vi "Main Tclk.vi"() -> ()   [LabVIEW 2018] (continued)
            n4337 = Index Array(array=w3502) -> (element #1=w3500:i32, element #2=w3499:i32)  [unwired: 2 in]
            n4338 = Bundle By Name(cluster=w3506, "Y stig"=w3501, "X tiles"=w3499, "Y tiles"=w3500) -> (w3505:T26)
            n4339 = local write "SEM Scan Parameters"(w3505) -> ()
          }
          event "SEM Scan Parameters.X aln": Mouse Down; "SEM Scan Parameters.X aln": Value Change {
            n4340 = event-data() -> ()  [unwired: 5 out]
            n4341 = local read "SEM Scan Parameters"() -> (w3518:T26)
            n4342 = Unbundle By Name(w3518) -> ("X aln"=w3520:sgl[][], "X tiles"=w3516:u8, "Y tiles"=w3515:u8)
            n4343 = call "2D array edit.vi"("Data Entry Limits:Increment"=0.1, "Display Format:Precision"=u8 2, "Rows"=w3515, "Columns"=w3516, "Caption.Text"="X aln (%)", "Input array"=w3520) -> ("Output array"=w3513:sgl[][])  [unwired: 5 in]
            n4344 = Array Size(array=w3513) -> (size(s)=w3514:i32[])
            n4345 = Index Array(array=w3514) -> (element #1=w3512:i32, element #2=w3511:i32)  [unwired: 2 in]
            n4346 = Bundle By Name(cluster=w3518, "X aln"=w3513, "X tiles"=w3511, "Y tiles"=w3512) -> (w3517:T26)
            n4347 = local write "SEM Scan Parameters"(w3517) -> ()
          }
          event "SEM Scan Parameters.Y aln": Mouse Down; "SEM Scan Parameters.Y aln": Value Change {
            n4348 = event-data() -> ()  [unwired: 5 out]
            n4349 = local read "SEM Scan Parameters"() -> (w3530:T26)
            n4350 = Unbundle By Name(w3530) -> ("Y aln"=w3532:sgl[][], "X tiles"=w3528:u8, "Y tiles"=w3527:u8)
            n4351 = call "2D array edit.vi"("Data Entry Limits:Increment"=0.1, "Display Format:Precision"=u8 2, "Rows"=w3527, "Columns"=w3528, "Caption.Text"="Y aln (%)", "Input array"=w3532) -> ("Output array"=w3525:sgl[][])  [unwired: 5 in]
            n4352 = Array Size(array=w3525) -> (size(s)=w3526:i32[])
            n4353 = Index Array(array=w3526) -> (element #1=w3523:i32, element #2=w3524:i32)  [unwired: 2 in]
            n4354 = Bundle By Name(cluster=w3530, "Y aln"=w3525, "X tiles"=w3524, "Y tiles"=w3523) -> (w3529:T26)
            n4355 = local write "SEM Scan Parameters"(w3529) -> ()
          }
          event "SEM Scan Parameters.dX (um)": Mouse Down {
            w3535 = u8 1 ("Rows")
            n4356 = event-data() -> ()  [unwired: 9 out]
            n4357 = local read "SEM Scan Parameters"() -> (w3543:T26)
            n4358 = local write "Delta X array for stop limit"(sgl[] [] ("Delta X array for stop limit")) -> ()
            n4359 = Unbundle By Name(w3543) -> ("dX (um)"=w3539:sgl[], "Y tiles"=w3534:u8)
            n4360 = Reshape Array(w3539, w3534, w3535) -> (w3538:sgl[][])
            n4361 = call "2D array edit.vi"("Data Entry Limits:Increment"=0.1, "Display Format:Precision"=u8 2, "Rows"=w3534, "Columns"=w3535, "Caption.Text"="dX (um)", "Input array"=w3538) -> ("Output array"=w3537:sgl[][])  [unwired: 5 in]
            n4362 = Reshape Array(w3537, w3534) -> (w3536:sgl[])
            n4363 = Bundle By Name(cluster=w3543, "dX (um)"=w3536, "Y tiles"=w3534) -> (w3542:T26)
            n4364 = local write "SEM Scan Parameters"(w3542) -> ()
          }
          event "SEM Scan Parameters.dY (um)": Mouse Down {
            w3550 = u8 1 ("Rows")
            n4365 = event-data() -> ()  [unwired: 9 out]
            n4366 = local read "SEM Scan Parameters"() -> (w3555:T26)
            n4367 = local write "Delta Y array for stop limit"(sgl[] [] ("Delta X array for stop limit")) -> ()
            n4368 = Unbundle By Name(w3555) -> ("dY (um)"=w3551:sgl[], "X tiles"=w3546:u8)
            n4369 = Reshape Array(w3551, w3550, w3546) -> (w3549:sgl[][])
            n4370 = call "2D array edit.vi"("Data Entry Limits:Increment"=0.1, "Display Format:Precision"=u8 2, "Rows"=w3550, "Columns"=w3546, "Caption.Text"="dY (um)", "Input array"=w3549) -> ("Output array"=w3548:sgl[][])  [unwired: 5 in]
            n4371 = Reshape Array(w3548, w3546) -> (w3547:sgl[])
            n4372 = Bundle By Name(cluster=w3555, "dY (um)"=w3547, "X tiles"=w3546) -> (w3554:T26)
            n4373 = local write "SEM Scan Parameters"(w3554) -> ()
          }
          event "Mid Mag SEM": Value Change {
            n4374 = event-data() -> ()  [unwired: 6 out]
          }
          event "Mill Manual Pause": Value Change {
            w3562 = u8 0 ("AF Count")
            w3564 = FALSE ("Reset WD")
            w3563 = TRUE ("Reset WD")
            n4375 = event-data() -> ("NewVal"=w3565:bool)  [unwired: 5 out]
            n4376 = case shown="False" w3565 {
              frame False {
                n4377 = local read "Status message"() -> (w3571:string)
                n4378 = Equal?(x=w3571, y="Manual pausing ..." ("Status message")) -> (x = y?=w3570:bool)
                n4379 = Select(t="SEM between FIB" ("Status message"), s=w3570, f="Resume FIB milling ..." ("Status message")) -> (s? t:f=w3569:string)
                n4380 = local write "Status message"(w3569) -> ()
              }
              frame True {
                n4381 = local read "Status message"() -> (w3577:string)
                n4382 = Equal?(x=w3577, y="SEM between FIB" ("Status message")) -> (x = y?=w3574:bool)
                n4383 = Select(t="Manual pausing ..." ("Status message"), s=w3574, f="Manual paused" ("Status message")) -> (s? t:f=w3573:string)
                n4384 = local write "Status message"(w3573) -> ()
              }
            }
            n4385 = local write "SW error warning armed"(w3563) -> ()
            n4386 = local write "Auto Focus"(w3564) -> ()
            n4387 = local write "Auto Stig"(w3564) -> ()
            n4388 = local write "Auto Align"(w3564) -> ()
            n4389 = local write "Reset Focus"(w3563) -> ()
            n4390 = local write "3D image paused armed"(w3563) -> ()
            n4391 = local write "Temperature warning armed"(w3563) -> ()
            n4392 = local write "AF Count"(w3562) -> ()
            n4393 = local write "AS Count"(w3562) -> ()
            n4394 = local write "AA Count"(w3562) -> ()
            n4395 = local read "SEM Scan Parameters"() -> (w3558:T26)
            n4396 = Unbundle By Name(w3558) -> ("Y tiles"=w3559:u8, "X tiles"=w3560:u8)
            n4397 = Initialize Array(FALSE ("ASX Success"), w3559, w3560) -> (w3561:bool[][])
            n4398 = local write "AAY Success tiled"(w3561) -> ()
            n4399 = local write "AF Success tiled"(w3561) -> ()
            n4400 = local write "ASX Success tiled"(w3561) -> ()
            n4401 = local write "ASY Success tiled"(w3561) -> ()
            n4402 = local write "AAX Success tiled"(w3561) -> ()
          }
          event "Save Probe Table": Value Change {
            n4403 = event-data() -> ("NewVal"=w3578:bool)  [unwired: 5 out]
            n4404 = case shown="True" w3578 {
              frame False {
              }
              frame True {
                n4405 = Two Button Dialog(message="Save FIB Probe Table?") -> (T button?=w3579:bool)  [unwired: 2 in]
                n4406 = case shown="True" w3579 {
                  frame False {
                    n4407 = local write "Save Probe Table"(FALSE ("Min FIB probe")) -> ()
                  }
                  frame True {
                    n4408 = stacked-sequence {
                      frame #0 {
                        n4409 = local read "Api"() -> (w3583:refnum<k7>)
                        n4410 = local read "FIB Milling Probe"() -> (w3582:string)
                        n4411 = call "SmartSEM Remote API save FIB probe table.vi"("FIB Probe"=w3582, "Api"=w3583) -> ()  [unwired: 8 in, 2 out]
                        n4412 = local write "Status message"("Measuring FIB probe currents" ("Status message")) -> ()
                      }
                      frame #1 {
                        n4413 = local write "Save Probe Table"(FALSE ("Min FIB probe")) -> ()
                        n4414 = local write "Status message"("FIB Probe Table saved" ("Status message")) -> ()
                      }
                    }
                  }
                }
              }
            }
          }
          event "FIB Milling Probe": Value Change {
            n4415 = event-data() -> ()  [unwired: 6 out]
            n4416 = local read "Machine Type"() -> (w3587:u8)
            n4417 = case shown="2" w3587 {
              frame 0, Default {
              }
              frame 2 {
                n4418 = local read "Api"() -> (w3594:refnum<k7>)
                n4419 = call "SmartSEM Remote API set string.vi"("vValue"="FIB Milling Probe", "lpszParam"="DP_FIB_IMAGE_PROBE", "Api"=w3594) -> ("error out"=w3588:errorcluster, "Api out"=w3591:refnum<k7>)  [unwired: 7 in]
                n4420 = call "SmartSEM Remote API set string.vi"("error in"=w3588, "vValue"="Undefined", "lpszParam"="DP_FIB_MILL_PROBE", "Api"=w3591) -> ()  [unwired: 6 in, 2 out]
              }
            }
          }
          event "Min FIB probe": Value Change {
            n4421 = event-data() -> ("NewVal"=w3595:bool)  [unwired: 5 out]
            n4422 = case shown="True" w3595 {
              frame False {
              }
              frame True {
                n4423 = Two Button Dialog(message="Switch to min current of the same probe size?") -> (T button?=w3596:bool)  [unwired: 2 in]
                n4424 = case shown="True" w3596 {
                  frame False {
                    n4425 = local write "Min FIB probe"(FALSE ("Min FIB probe")) -> ()
                  }
                  frame True {
                    n4426 = stacked-sequence {
                      frame #0 {
                        n4427 = local read "Api"() -> (w3601:refnum<k7>)
                        n4428 = local read "FIB Milling Probe"() -> (w3602:string)
                        n4429 = local write "Min FIB probe"(FALSE ("Min FIB probe")) -> ()
                        n4430 = call "SmartSEM Remote API goto min or max FIB probe current.vi"("Min or Max"="Min", "FIB Probe"=w3602, "Api"=w3601) -> ("Goto probe"=w3599:string)  [unwired: 7 in, 1 out]
                        n4431 = local write "FIB Milling Probe"(w3599) -> ()
                        n4432 = local write "Status message"("Measuring FIB probe currents" ("Status message")) -> ()
                      }
                      frame #1 {
                        n4433 = local write "Status message"("Switched to minimal current of the same probe" ("Status message")) -> ()
                      }
                    }
                  }
                }
              }
            }
          }
          event "Max FIB probe": Value Change {
            n4434 = event-data() -> ("NewVal"=w3606:bool)  [unwired: 5 out]
            n4435 = case shown="True" w3606 {
              frame False {
              }
              frame True {
                n4436 = Two Button Dialog(message="Switch to max current of the same probe size?") -> (T button?=w3607:bool)  [unwired: 2 in]
                n4437 = case shown="True" w3607 {
                  frame False {
                    n4438 = local write "Max FIB probe"(FALSE ("Min FIB probe")) -> ()
                  }
                  frame True {
                    n4439 = stacked-sequence {
                      frame #0 {
                        n4440 = local read "Api"() -> (w3613:refnum<k7>)
                        n4441 = local read "FIB Milling Probe"() -> (w3612:string)
                        n4442 = local write "Max FIB probe"(FALSE ("Min FIB probe")) -> ()
                        n4443 = call "SmartSEM Remote API goto min or max FIB probe current.vi"("Min or Max"="Max", "FIB Probe"=w3612, "Api"=w3613) -> ("Goto probe"=w3611:string)  [unwired: 7 in, 1 out]
                        n4444 = local write "FIB Milling Probe"(w3611) -> ()
                        n4445 = local write "Status message"("Measuring FIB probe currents" ("Status message")) -> ()
                      }
                      frame #1 {
                        n4446 = local write "Status message"("Switched to maximal current of the same probe" ("Status message")) -> ()
                      }
                    }
                  }
                }
              }
            }
          }
          event "FIB time lapse": Value Change {
            n4447 = event-data() -> ("NewVal"=w3617:bool)  [unwired: 5 out]
            n4448 = case shown="False" w3617 {
              frame False {
                n4449 = stacked-sequence {
                  frame #0 {
                    n4450 = local read "FIB HW Config"() -> (w3620:T23)
                    n4451 = Unbundle By Name(w3620) -> ("Beam blank"=w3621:tag)
                    n4452 = local read "Api"() -> (w3618:refnum<k7>)
                    n4453 = call "FIB beam blank.vi"("Api"=w3618, "Beam blanked"=TRUE ("Ext on"), "lines"=w3621) -> ()  [unwired: 2 in, 1 out]
                  }
                  frame #1 {
                    n4454 = local read "SEM HW Config"() -> (w3626:T9)
                    n4455 = Unbundle By Name(w3626) -> ("Detector FIB-NI auto switch"=w3627:tag)
                    n4456 = call-poly <vilib>:"DAQmx Create Virtual Channel.vi"("lines"=w3627) -> ("task out"=w3624:refnum<k21>, "error out"=w3625:errorcluster)  [unwired: 4 in, 9 out]
                    n4457 = call-poly <vilib>:"DAQmx Write.vi"("task/channels in"=w3624, "data"=FALSE, "error in"=w3625) -> ("task out"=w3622:refnum<k21>, "error out"=w3623:errorcluster)  [unwired: 1 in, 10 out]
                    n4458 = call <vilib>:"DAQmx Clear Task.vi"("task in"=w3622, "error in"=w3623) -> ()  [unwired: 14 out]
                  }
                  frame #2 {
                    n4459 = local read "FIB HW Config"() -> (w3631:T23)
                    n4460 = Unbundle By Name(w3631) -> ("FIB Ext Scan"=w3630:tag)
                    n4461 = call "FIB ext scan.vi"("Ext on"=FALSE, "FIB Ext Scan"=w3630) -> ()  [unwired: 9 in, 1 out]
                  }
                  frame #3 {
                    n4462 = local read "Machine Type"() -> (w3632:u8)
                    n4463 = case shown="2" w3632 {
                      frame 0, Default {
                      }
                      frame 1 {
                        w3633 = TRUE ("Initialization")
                        n4464 = local read "COM port"() -> (w3639:refnum<visa-resource-name>)
                        n4465 = call "FIB mode.vi"("Initialization"=w3633, "FIB mode"=T10."SEM", "COM port in"=w3639) -> ("COM port out"=w3638:refnum<visa-resource-name>)  [unwired: 7 in, 1 out]
                        n4466 = call "Remcon32 command.vi"("SEM command"="edx 0", "COM port in"=w3638) -> ("COM port out"=w3637:refnum<visa-resource-name>)  [unwired: 6 in, 3 out]
                        n4467 = call "Remcon32 command.vi"("Close session"=w3633, "SEM command"="frez", "COM port in"=w3637) -> ()  [unwired: 5 in, 4 out]
                      }
                      frame 2 {
                        n4468 = local read "Api"() -> (w3640:refnum<k7>)
                        n4469 = call "SmartSEM Remote API set float.vi"("vValue"=sgl 2.0, "lpszParam"="DP_FIB_BLANKER_MODE" ("lpszCommand"), "Api"=w3640) -> ("error out"=w3641:errorcluster, "Api out"=w3642:refnum<k7>)  [unwired: 7 in]
                        n4470 = call "SmartSEM Remote API FIB mode.vi"("error in"=w3641, "FIB mode"=T50."SEM", "Api"=w3642) -> ("error out"=w3645:errorcluster, "Api out"=w3646:refnum<k7>)  [unwired: 7 in]
                        n4471 = invoke class="_EMApi" method="Execute"(reference=w3646, error in=w3645, "lpszCommand"="CMD_FREEZE_ALL") -> ()  [unwired: 1 in, 4 out]
                      }
                    }
                  }
                  frame #4 {
                    n4472 = local write "Status message"("standby" ("Status message")) -> ()
                  }
                }
              }
              frame True {
              }
            }
          }
          event "FIB Image": Mouse Down {
            n4473 = event-data() -> ("Coords"=→"Mouse Down Coords":T22)  [unwired: 3 out]
            n4474 = register-events(reference=w3658, w3654) -> (reference out=w3657:refnum<event-registration>, error out=w3656:errorcluster)  [unwired: 1 in]
            n4475 = local read "Spot"() -> (w3653:bool)
            n4476 = property on="Cursor Z (V)" class="DigNum (strict)"("Visible"=FALSE) -> ()  [unwired: 2 in, 2 out]
            n4477 = case shown="True" w3653 {
              frame False {
              }
              frame True {
                n4478 = local read "FIB HW Config"() -> (w3662:T23)
                n4479 = Unbundle By Name(w3662) -> ("Beam blank"=w3661:tag)
                n4480 = local read "Api"() -> (w3659:refnum<k7>)
                n4481 = call "FIB beam blank.vi"("Api"=w3659, "Beam blanked"=TRUE, "lines"=w3661) -> ()  [unwired: 2 in, 1 out]
              }
            }
            "Mouse down" <- TRUE ("Mouse down")
          }
          event "FIB Image": Mouse Move {
            n4482 = event-data() -> ("Coords"=w3667:T22)  [unwired: 1 out]
            n4483 = local read "Mouse down"() -> (w3666:bool)
            n4484 = local read "Spot"() -> (w3665:bool)
            n4485 = local read "FIB"() -> (w3664:bool)
            n4486 = Or(x=w3665, y=w3664) -> (x .or. y?=w3663:bool)
            n4487 = case shown="False" w3666 {
              tunnel: [w3694 w3698] -> w3669
              tunnel: w3668 -> [w3694 w3697]
              tunnel: w3667 -> [w3693 w3696]
              tunnel: w3663 -> [_ w3695]
              frame False {
                w3670 = i16 0 ("upper limit")
                n4488 = property on="FIB Image" class="IntGraph (strict)"() -> ("Plot Bounds"=w3692:T71, "Width"=w3674:u32, "Height"=w3682:u32)  [unwired: 2 in, 2 out]
                n4489 = local read "FIB Scan Parameters"() -> (w3691:T32)
                n4490 = Unbundle By Name(w3692) -> ("Right"=w3677:i16, "Bottom"=w3685:i16)
                n4491 = Unbundle By Name(w3693) -> ("Horizontal"=w3676:i32, "Vertical"=w3678:i32)
                n4492 = Unbundle By Name(w3691) -> ("Z size (V)"=w3684:dbl)
                n4493 = To Word Integer(number=w3682) -> (16bit integer=w3680:i16)
                n4494 = To Word Integer(number=w3678) -> (16bit integer=w3679:i16)
                n4495 = Subtract(x=w3677, y=w3676) -> (x-y=w3675:i32)
                n4496 = Subtract(x=w3685, y=w3679) -> (x-y=w3681:i16)
                n4497 = In Range and Coerce(upper limit=w3674, x=w3675, lower limit=w3670) -> (In Range?=w3673:bool)  [unwired: 1 out]
                n4498 = In Range and Coerce(upper limit=w3680, x=w3681, lower limit=w3670) -> (coerced(x)=w3683:i16, In Range?=w3672:bool)
                n4499 = Multiply(x=w3683, y=w3684) -> (x*y=w3690:dbl)
                n4500 = Multiply(x=w3684, y=0.5) -> (x*y=w3688:dbl)
                n4501 = And(x=w3673, y=w3672) -> (x .and. y?=w3671:bool)
                n4502 = Divide(x=w3690, y=w3682) -> (x/y=w3689:dbl)
                n4503 = property on="Cursor Z (V)" class="DigNum (strict)"("Visible"=w3671) -> ()  [unwired: 2 in, 2 out]
                n4504 = Subtract(x=w3689, y=w3688) -> (x-y=→"Cursor Z (V)":dbl)
              }
              frame True {
                n4505 = case shown="False" w3695 {
                  tunnel: w3696 -> [w3700 _]
                  tunnel: [w3699 w3823] -> w3698
                  tunnel: w3697 -> [_ w3823]
                  frame False {
                    n4506 = stacked-sequence {
                      tunnel: w3700 -> [_ w3705]
                      tunnel: [_ w3703] -> w3699
                      frame #0 {
                        n4507 = call <vilib>:"Draw Rectangle.vi"("picture"=picture data[5B]) -> ("new picture"=w3702:picture)  [unwired: 8 in]
                        n4508 = property on="FIB Image" class="IntGraph (strict)"("PlotImages.Front"=w3702) -> ()  [unwired: 2 in, 2 out]
                      }
                      frame #1 {
                        n4509 = case shown="True" "ROI" {
                          tunnel: w3705 -> [w3747 w3814]
                          tunnel: [w3706 w3758] -> w3703
                          frame False {
                            w3724 = 5 ("dimension size")
                            w3745 = u32 16711680 ("color(black)")
                            n4510 = local read "Mouse Down Coords"() -> (w3748:T22)
                            n4511 = Subtract(x=w3747, y=w3748) -> (x-y=w3746:T22)
                            n4512 = Unbundle By Name(w3746) -> ("Horizontal"=w3725:i32, "Vertical"=w3723:i32)
                            n4513 = Initialize Array(w3725, w3724) -> (w3722:i32[])
                            n4514 = Initialize Array(w3723, w3724) -> (w3721:i32[])
                            n4515 = local read "FIB Scan Parameters"() -> (w3735:T32)
                            n4516 = local read "Milling para"() -> (w3740:T35)
                            n4517 = local read "FIB Options"() -> (w3741:T33)
                            n4518 = local read "Trapezoidal"() -> (w3707:cluster{"X":i16, "Y":i16}[])
                            n4519 = Build Cluster Array(w3722, w3721) -> (w3720:cluster{"Horizontal":i32, "Vertical":i32}[])
                            n4520 = To Word Integer(number=w3720) -> (16bit integer=w3719:cluster{"Horizontal":i16, "Vertical":i16}[])
                            n4521 = Unbundle By Name(w3740) -> ("Mill from Bottom"=w3739:bool)
                            n4522 = Unbundle By Name(w3741) -> ("Flip z"=w3727:bool)
                            n4523 = Add(x=w3719, y=w3707) -> (x+y=w3706:cluster{i16, i16}[])
                            n4524 = Unbundle By Name(w3735) -> ("Z size (V)"=w3736:dbl)
                            n4525 = for {
                              tunnel: w3706 -> [w3757] mode=indexing
                              tunnel: [w3756] -> w3718 mode=indexing
                              tunnel: [w3755] -> w3713 mode=indexing
                              n4526 = Unbundle(w3757) -> (w3756:i16, w3755:i16)
                            }
                            n4527 = Exclusive Or(1:w3727, 2:w3739) -> (0:w3710:bool)
                            n4528 = case shown="False" w3710 {
                              tunnel: [2 ("index") 0 ("index")] -> w3717
                              tunnel: [3 ("index") 1 ("index")] -> w3716
                              frame False {
                              }
                              frame True {
                              }
                            }
                            n4529 = Index Array(array=w3713, index #1=0 ("index"), index #2=2 ("index")) -> (element #1=w3712:i16, element #2=w3711:i16)
                            n4530 = Index Array(array=w3718, index #1=w3717, index #2=w3716) -> (element #1=w3708:i16, element #2=w3709:i16)
                            n4531 = Select(t=w3712, s=w3710, f=w3711) -> (s? t:f=w3726:i16)
                            n4532 = property on="FIB Image" class="IntGraph (strict)"() -> ("Height"=w3734:u32)  [unwired: 2 in, 2 out]
                            n4533 = Divide(x=w3726, y=w3734) -> (x/y=w3733:dbl)
                            n4534 = Subtract(x=w3733, y=0.5) -> (x-y=w3731:dbl)
                            n4535 = call <vilib>:"Draw Multiple Lines.vi"("picture"=picture data[5B], "line endpoints"=w3706, "color(black)"=u32 6618880) -> ("new picture"=w3744:picture)  [unwired: 6 in]
                            n4536 = Multiply(x=w3731, y=w3736) -> (x*y=w3730:dbl)
                            n4537 = Bundle(w3708, w3726) -> (w3738:cluster{i16, i16})  [unwired: 1 in]
                            n4538 = Bundle(w3709, w3726) -> (w3737:cluster{i16, i16})  [unwired: 1 in]
                            n4539 = Negate(x=w3730) -> (-x=w3729:dbl)
                            n4540 = call <vilib>:"Draw Point.vi"("picture"=w3744, "point(x,y)"=w3738, "color(black)"=w3745) -> ("new picture"=w3743:picture)  [unwired: 6 in]
                            n4541 = Select(t=w3729, s=w3727, f=w3730) -> (s? t:f=w3728:dbl)
                            n4542 = call <vilib>:"Draw Line.vi"("picture"=w3743, "end point"=w3737, "color(black)"=w3745) -> ("new picture"=w3742:picture)  [unwired: 6 in]
                            n4543 = shared-variable ".\\Zeiss Library.lvlib\\Milling Z Voltage RT"(w3728) -> ()  [unwired: 1 in, 1 out]
                            n4544 = property on="FIB Image" class="IntGraph (strict)"("PlotImages.Front"=w3742) -> ()  [unwired: 2 in, 2 out]
                          }
                          frame True {
                            w3794 = u32 16711680 ("color(black)")
                            w3798 = T46 {"left"=0, "top"=0, "right"=0, "bottom"=0} ("rect")
                            n4545 = local read "Mouse Down Coords"() -> (w3813:T22)
                            n4546 = property on="FIB Image" class="IntGraph (strict)"() -> ("Plot Bounds"=w3797:T71)  [unwired: 2 in, 2 out]
                            n4547 = Unbundle By Name(w3814) -> ("Horizontal"=w3812:i32, "Vertical"=w3810:i32)
                            n4548 = Unbundle By Name(w3813) -> ("Horizontal"=w3811:i32, "Vertical"=w3809:i32)
                            n4549 = local read "FIB Scan Parameters"() -> (w3787:T32)
                            n4550 = local read "Milling para"() -> (w3781:T35)
                            n4551 = local read "FIB Options"() -> (w3791:T33)
                            n4552 = Unbundle By Name(w3797) -> ("Left"=w3804:i16, "Top"=w3803:i16)
                            n4553 = Unbundle By Name(w3797) -> ("Left"=w3802:i16, "Top"=w3801:i16)
                            n4554 = Max & Min(x=w3812, y=w3811) -> (max(x,y)=w3808:i32, min(x,y)=w3807:i32)
                            n4555 = Max & Min(x=w3810, y=w3809) -> (max(x,y)=w3805:i32, min(x,y)=w3806:i32)
                            n4556 = Bundle By Name(cluster=w3798, "left"=w3807, "top"=w3806, "right"=w3808, "bottom"=w3805) -> (w3800:T46)
                            n4557 = Bundle By Name(cluster=w3798, "left"=w3804, "top"=w3803, "right"=w3802, "bottom"=w3801) -> (w3799:T46)
                            n4558 = Unbundle By Name(w3781) -> ("Mill from Bottom"=w3779:bool)
                            n4559 = Unbundle By Name(w3791) -> ("Flip z"=w3778:bool)
                            n4560 = Unbundle By Name(w3787) -> ("Z size (V)"=w3785:dbl)
                            n4561 = Subtract(x=w3800, y=w3799) -> (x-y=w3760:T46)
                            n4562 = Unbundle By Name(w3760) -> ("left"=w3776:i16, "top"=w3766:i16, "right"=w3773:i16, "bottom"=w3765:i16)
                            n4563 = Exclusive Or(1:w3778, 2:w3779) -> (0:w3777:bool)
                            n4564 = Select(t=w3766, s=w3777, f=w3765) -> (s? t:f=w3780:i16)
                            n4565 = property on="FIB Image" class="IntGraph (strict)"() -> ("Height"=w3790:u32)  [unwired: 2 in, 2 out]
                            n4566 = Initialize Array(w3776, 5 ("dimension size")) -> (w3774:i16[])
                            n4567 = Initialize Array(w3766, 5 ("dimension size")) -> (w3767:i16[])
                            n4568 = Divide(x=w3780, y=w3790) -> (x/y=w3789:dbl)
                            n4569 = Subtract(x=w3789, y=0.5) -> (x-y=w3786:dbl)
                            n4570 = Replace Array Subset(array=w3774, new element #1=w3773, index #1=1 ("index"), new element #2=w3773, index #2=2 ("index")) -> (w3764:i16[])
                            n4571 = Replace Array Subset(array=w3767, new element #1=w3765, index #1=2 ("index"), new element #2=w3765, index #2=3 ("index")) -> (w3763:i16[])
                            n4572 = Multiply(x=w3786, y=w3785) -> (x*y=w3784:dbl)
                            n4573 = Build Cluster Array(w3764, w3763) -> (w3758:cluster{"left":i16, "top":i16}[])
                            "Trapezoidal" <- w3758
                            n4574 = Negate(x=w3784) -> (-x=w3783:dbl)
                            n4575 = Select(t=w3783, s=w3778, f=w3784) -> (s? t:f=w3782:dbl)
                            n4576 = shared-variable ".\\Zeiss Library.lvlib\\Milling Z Voltage RT"(w3782) -> ()  [unwired: 1 in, 1 out]
                            n4577 = call <vilib>:"Draw Multiple Lines.vi"("picture"=picture data[5B], "line endpoints"=w3758, "color(black)"=u32 6618880) -> ("new picture"=w3759:picture)  [unwired: 6 in]
                            n4578 = Bundle("left"=w3776, "bottom"=w3780) -> (w3795:cluster{"left":i16, "bottom":i16})  [unwired: 1 in]
                            n4579 = Bundle("right"=w3773, "bottom"=w3780) -> (w3793:cluster{"right":i16, "bottom":i16})  [unwired: 1 in]
                            n4580 = call <vilib>:"Draw Point.vi"("picture"=w3759, "point(x,y)"=w3795, "color(black)"=w3794) -> ("new picture"=w3796:picture)  [unwired: 6 in]
                            n4581 = call <vilib>:"Draw Line.vi"("picture"=w3796, "end point"=w3793, "color(black)"=w3794) -> ("new picture"=w3792:picture)  [unwired: 6 in]
                            n4582 = property on="FIB Image" class="IntGraph (strict)"("PlotImages.Front"=w3792) -> ()  [unwired: 2 in, 2 out]
                          }
                        }
                      }
                    }
                  }
                  frame True {
                    w3819 = 1.0 ("upper limit")
                    w3820 = 511.0 ("upper limit")
                    w3821 = 0.0 ("Y Scale.Range:Minimum")
                    w3822 = 512.0 ("X Scale.Range:Maximum")
                    n4583 = property on="FIB Image" class="IntGraph (strict)"("XScale.Maximum"=w3822, "XScale.Minimum"=w3821, "YScale.Maximum"=w3822, "YScale.Minimum"=w3821) -> ("Cursor.Cursor X"=w3818:dbl, "Cursor.Cursor Y"=w3817:dbl)  [unwired: 2 in, 2 out]
                    n4584 = In Range and Coerce(upper limit=w3820, x=w3818, lower limit=w3819) -> (coerced(x)=w3816:dbl)  [unwired: 1 out]
                    n4585 = In Range and Coerce(upper limit=w3820, x=w3817, lower limit=w3819) -> (coerced(x)=w3815:dbl)  [unwired: 1 out]
                    n4586 = property on="FIB Image" class="IntGraph (strict)"("Cursor.Cursor X"=w3816, "Cursor.Cursor Y"=w3815) -> ()  [unwired: 2 in, 2 out]
                  }
                }
              }
            }
          }
          event "FIB Image": Mouse Up {
            w3828 = i16 0 ("upper limit")
            n4587 = event-data() -> ("Coords"=w3827:T22)  [unwired: 3 out]
            n4588 = local read "Mouse Down Coords"() -> (w3857:T22)
            n4589 = property on="FIB Image" class="IntGraph (strict)"() -> ("Plot Bounds"=w3849:T71, "Width"=w3832:u32, "Height"=w3840:u32)  [unwired: 2 in, 2 out]
            n4590 = local read "FIB Scan Parameters"() -> (w3848:T32)
            n4591 = Equal?(x=w3857, y=w3827) -> (x = y?=w3856:cluster{"Horizontal":bool, "Vertical":bool})
            n4592 = Unbundle By Name(w3849) -> ("Right"=w3835:i16, "Bottom"=w3843:i16)
            n4593 = Unbundle By Name(w3827) -> ("Horizontal"=w3834:i32, "Vertical"=w3836:i32)
            n4594 = Unbundle By Name(w3856) -> ("Horizontal"=w3854:bool, "Vertical"=w3855:bool)
            n4595 = register-events(reference=w3861, refnum<k0> refnum) -> (reference out=w3860:refnum<event-registration>, error out=w3859:errorcluster)  [unwired: 1 in]
            n4596 = local write "Mouse down"(FALSE ("Mouse down")) -> ()
            n4597 = local read "Spot"() -> (w3824:bool)
            n4598 = local read "FIB"() -> (w3853:bool)
            n4599 = Unbundle By Name(w3848) -> ("Z size (V)"=w3842:dbl)
            n4600 = To Word Integer(number=w3840) -> (16bit integer=w3838:i16)
            n4601 = To Word Integer(number=w3836) -> (16bit integer=w3837:i16)
            n4602 = Subtract(x=w3835, y=w3834) -> (x-y=w3833:i32)
            n4603 = Subtract(x=w3843, y=w3837) -> (x-y=w3839:i16)
            n4604 = And(x=w3854, y=w3855) -> (x .and. y?=w3852:bool)
            n4605 = In Range and Coerce(upper limit=w3832, x=w3833, lower limit=w3828) -> (In Range?=w3831:bool)  [unwired: 1 out]
            n4606 = In Range and Coerce(upper limit=w3838, x=w3839, lower limit=w3828) -> (coerced(x)=w3841:i16, In Range?=w3830:bool)
            n4607 = Compound Arithmetic op=OR(w3824, w3853, w3852) -> (w3851:bool)
            n4608 = Multiply(x=w3841, y=w3842) -> (x*y=w3847:dbl)
            n4609 = Multiply(x=w3842, y=0.5) -> (x*y=w3845:dbl)
            n4610 = And(x=w3831, y=w3830) -> (x .and. y?=w3829:bool)
            n4611 = Divide(x=w3847, y=w3840) -> (x/y=w3846:dbl)
            n4612 = property on="Cursor Z (V)" class="DigNum (strict)"("Visible"=w3829) -> ()  [unwired: 2 in, 2 out]
            n4613 = Subtract(x=w3846, y=w3845) -> (x-y=w3826:dbl)
            n4614 = local write "Cursor Z (V)"(w3826) -> ()
            n4615 = case shown="True" w3851 {
              tunnel: w3825 -> [w3867 _]
              tunnel: w3824 -> [_ w3934]
              frame False {
                n4616 = for {
                  tunnel: w3867 -> [w3925] mode=indexing
                  tunnel: [w3924] -> w3901 mode=indexing
                  tunnel: [w3923] -> w3878 mode=indexing
                  n4617 = Unbundle(w3925) -> ("X"=w3924:i16, "Y"=w3923:i16)
                }
                n4618 = local write "Trapezoidal"(w3867) -> ()
                n4619 = property on="FIB Image" class="IntGraph (strict)"() -> ("Height"=w3877:u32, "Width"=w3890:u32)  [unwired: 2 in, 2 out]
                n4620 = Divide(x=w3877, y=w3890) -> (x/y=w3918:dbl)
                n4621 = Index Array(array=w3901, index #1=1 ("index"), index #2=2 ("index"), index #3=0 ("index"), index #4=3 ("index")) -> (element #1=w3871:i16, element #2=w3872:i16, element #3=w3873:i16, element #4=w3898:i16)
                n4622 = Index Array(array=w3878, index #1=2 ("index"), index #2=3 ("index"), index #3=0 ("index"), index #4=1 ("index")) -> (element #1=w3868:i16, element #2=w3869:i16, element #3=w3870:i16, element #4=w3883:i16)
                n4623 = local read "Milling para"() -> (w3920:T35)
                n4624 = Add(x=w3871, y=w3872) -> (x+y=w3897:i16)
                n4625 = Add(x=w3873, y=w3898) -> (x+y=w3896:i16)
                n4626 = Add(x=w3868, y=w3869) -> (x+y=w3884:i16)
                n4627 = Add(x=w3870, y=w3883) -> (x+y=w3885:i16)
                n4628 = expression code="x*2"(w3890) -> (w3894:u32)
                n4629 = expression code="x*2"(w3877) -> (w3887:u32)
                n4630 = Unbundle By Name(w3920) -> ("FIB FOV (um)"=w3919:sgl, "Z-step (nm)"=w3862:dbl)
                n4631 = Add(x=w3897, y=w3896) -> (x+y=w3895:i16)
                n4632 = Subtract(x=w3897, y=w3896) -> (x-y=w3891:i16)
                n4633 = Add(x=w3884, y=w3885) -> (x+y=w3886:i16)
                n4634 = Subtract(x=w3884, y=w3885) -> (x-y=w3889:i16)
                n4635 = Divide(x=w3895, y=w3894) -> (x/y=w3893:dbl)
                n4636 = Divide(x=w3891, y=w3890) -> (x/y=w3875:dbl)
                n4637 = Divide(x=w3886, y=w3887) -> (x/y=w3888:dbl)
                n4638 = Divide(x=w3889, y=w3877) -> (x/y=w3874:dbl)
                n4639 = Decrement(x=w3893) -> (x-1=w3892:dbl)
                n4640 = Decrement(x=w3888) -> (x-1=w3876:dbl)
                n4641 = expression code="x/2"(w3919) -> (w3908:sgl)
                n4642 = expression code="x/1e3"(w3862) -> (w3907:dbl)
                n4643 = Compound Arithmetic op=MULTIPLY(w3874, w3908, w3918) -> (w3917:dbl)
                n4644 = Divide(x=w3917, y=w3907) -> (x/y=w3916:dbl)
                n4645 = Round To Nearest(number=w3916) -> (nearest integer value=w3904:dbl)
                n4646 = Multiply(x=w3892, y=w3908) -> (x*y=w3909:dbl)
                n4647 = Multiply(x=w3876, y=w3908) -> (x*y=w3910:dbl)
                n4648 = Multiply(x=w3875, y=w3908) -> (x*y=w3911:dbl)
                n4649 = Multiply(x=w3904, y=w3907) -> (x*y=w3906:dbl)
                n4650 = Round To Nearest(number=w3909) -> (nearest integer value=w3866:dbl)
                n4651 = Round To Nearest(number=w3910) -> (nearest integer value=w3865:dbl)
                n4652 = expression code="log2( x/0.1)"(w3911) -> (w3913:dbl)
                n4653 = Round To Nearest(number=w3911) -> (nearest integer value=w3864:dbl)
                n4654 = Round To Nearest(number=w3906) -> (nearest integer value=w3863:dbl)
                n4655 = Round Toward +Infinity(x=w3913) -> (ceil(x): smallest int >= x=w3915:dbl)
                n4656 = Increment(x=w3904) -> (x+1=w3905:dbl)
                n4657 = Scale By Power Of 2(n=w3915, x=ext 1.0) -> (x*2^n=w3912:ext)
                n4658 = local read "Milling para"() -> (w3921:T35)
                n4659 = Bundle By Name(cluster=w3921, "X center (um)"=w3866, "Z center (um)"=w3865, "X size (um)"=w3864, "Z size (um)"=w3863, "Z resolution"=w3905, "X resolution"=w3912) -> (w3922:T35)
                n4660 = local write "Milling para"(w3922) -> ()
              }
              frame True {
                w3928 = 1.0 ("upper limit")
                w3929 = 511.0 ("upper limit")
                w3932 = 0.0 ("Y Scale.Range:Minimum")
                w3933 = 512.0 ("X Scale.Range:Maximum")
                n4661 = case shown="True" w3934 {
                  frame False {
                  }
                  frame True {
                    n4662 = local read "FIB HW Config"() -> (w3938:T23)
                    n4663 = Unbundle By Name(w3938) -> ("Beam blank"=w3937:tag)
                    n4664 = local read "Api"() -> (w3935:refnum<k7>)
                    n4665 = call "FIB beam blank.vi"("Api"=w3935, "Beam blanked"=FALSE, "lines"=w3937) -> ()  [unwired: 2 in, 1 out]
                  }
                }
                n4666 = property on="FIB Image" class="IntGraph (strict)"("XScale.Maximum"=w3933, "XScale.Minimum"=w3932, "YScale.Maximum"=w3933, "YScale.Minimum"=w3932) -> ("Cursor.Cursor X"=w3931:dbl, "Cursor.Cursor Y"=w3930:dbl)  [unwired: 2 in, 2 out]
                n4667 = In Range and Coerce(upper limit=w3929, x=w3931, lower limit=w3928) -> (coerced(x)=w3927:dbl)  [unwired: 1 out]
                n4668 = In Range and Coerce(upper limit=w3929, x=w3930, lower limit=w3928) -> (coerced(x)=w3926:dbl)  [unwired: 1 out]
                n4669 = property on="FIB Image" class="IntGraph (strict)"("Cursor.Cursor X"=w3927, "Cursor.Cursor Y"=w3926) -> ()  [unwired: 2 in, 2 out]
              }
            }
          }
          event "SEM Shutter": Value Change {
            n4670 = event-data() -> ("NewVal"=w3943:bool)  [unwired: 1 out]
            n4671 = local read "Post #1up"() -> (w3942:tag)
            n4672 = local read "Post #1down"() -> (w3941:tag)
            n4673 = local read "Post #2up"() -> (w3940:tag)
            n4674 = local read "Post #2down"() -> (w3939:tag)
            n4675 = call "SEM shutter.vi"("Shutter close"=w3943, "Shutter AO4"=w3939, "Shutter AO3"=w3940, "Shutter AO2"=w3941, "Shutter AO1"=w3942) -> ()  [unwired: 6 in, 1 out]
          }
          event "FIB Profile": Value Change {
            n4676 = event-data() -> ("NewVal"=w3944:bool)  [unwired: 1 out]
            n4677 = case shown="True" w3944 {
              frame False {
              }
              frame True {
                n4678 = Two Button Dialog(message="Characterize FIB Beam Profile?") -> (T button?=w3945:bool)  [unwired: 2 in]
                n4679 = case shown="True" w3945 {
                  frame False {
                    n4680 = local write "FIB Profile"(FALSE ("FIB Profile")) -> ()
                  }
                  frame True {
                    n4681 = stacked-sequence {
                      frame #0 {
                        n4682 = local read "Enable logging"() -> (→"Logging status before profiling":bool)
                      }
                      frame #1 {
                        n4683 = local write "Enable logging"(FALSE ("Enable logging")) -> ()
                        n4684 = Wait (ms)(milliseconds to wait=u32 200) -> ()  [unwired: 1 out]
                        n4685 = local write "Image Tabs"(T37."Logging: Realtime Graphs" ("Image Tabs")) -> ()
                      }
                      frame #2 {
                        n4686 = local read "Machine Type"() -> (w3952:u8)
                        n4687 = case shown="2" w3952 {
                          frame 0, Default {
                            n4688 = local read "HV Data Output"() -> (w3957:T18)
                            n4689 = local read "FIB HW Config"() -> (w3965:T23)
                            n4690 = local read "FIB Options"() -> (w3963:T33)
                            n4691 = local read "Milling para"() -> (w3964:T35)
                            n4692 = local read "FIB Scan Parameters"() -> (w3967:T32)
                            n4693 = local read "Parameter Names"() -> (w3960:string[])
                            n4694 = Bundle By Name(cluster=w3967, "Frame line rampdown ratio"=0.0, "Oversampling"=u16 5) -> (w3962:T32)
                            n4695 = local read "Active logging channels"() -> (w3961:string)
                            n4696 = call "FIB profile.vi"("HV Data Output"=w3957, "Parameter Names"=w3960, "Active logging channels"=w3961, "Scan Para"=w3962, "Milling para"=w3964, "Options"=w3963, "HW Config"=w3965) -> ("Measurements"=w3959:dbl[][])  [unwired: 2 in, 2 out]
                            n4697 = local write "Measurements"(w3959) -> ()
                          }
                          frame 2 {
                            n4698 = local read "FIB HW Config"() -> (w3976:T23)
                            n4699 = local read "FIB Options"() -> (w3974:T33)
                            n4700 = local read "Milling para"() -> (w3975:T35)
                            n4701 = local read "FIB Scan Parameters"() -> (w3978:T32)
                            n4702 = local read "Parameter Names"() -> (w3971:string[])
                            n4703 = local read "Capella HV Data Output"() -> (w3968:T17)
                            n4704 = Bundle By Name(cluster=w3978, "Frame line rampdown ratio"=0.0, "Oversampling"=u16 5) -> (w3973:T32)
                            n4705 = local read "Active logging channels"() -> (w3972:string)
                            n4706 = call "FIB profile.vi"("Capella HV Data Output"=w3968, "Parameter Names"=w3971, "Active logging channels"=w3972, "Scan Para"=w3973, "Milling para"=w3975, "Options"=w3974, "HW Config"=w3976) -> ("Measurements"=w3970:dbl[][])  [unwired: 2 in, 2 out]
                            n4707 = local write "Measurements"(w3970) -> ()
                          }
                        }
                        n4708 = local write "Status message"("Scanning FIB vertically to obtain beam profile" ("Status message")) -> ()
                        n4709 = Get Date/Time In Seconds() -> (seconds since 1Jan1904=w3955:timestamp)
                        n4710 = To Double Precision Float(number=w3955) -> (double precision float=w3954:dbl)
                        n4711 = property on="Measurements" class="WFChart (strict)"("History Data"=dbl[][] [], "XScale.Offset"=w3954) -> ()  [unwired: 2 in, 2 out]
                        n4712 = call "Wait to resume.vi"() -> ()  [unwired: 12 in]
                      }
                      frame #3 {
                        n4713 = local read "Logging status before profiling"() -> (w3979:bool)
                        n4714 = local write "FIB Profile"(FALSE ("FIB Profile")) -> ()
                        n4715 = local write "Enable logging"(w3979) -> ()
                      }
                    }
                  }
                }
              }
            }
          }
          event "Milling para": Value Change {
            n4716 = event-data() -> ()  [unwired: 2 out]
            n4717 = local read "Milling para"() -> (w3995:T35)
            n4718 = local read "FIB"() -> (w4001:bool)
            n4719 = case shown="False" w4001 {
              tunnel: [TRUE ("Origin") FALSE ("Origin")] -> w4002
              tunnel: [0.0 ("Y offset pre (um)") w4018] -> w4000
              frame False {
              }
              frame True {
                n4720 = local read "Y offset pre (um)"() -> (w4018:dbl)
              }
            }
            n4721 = Unbundle By Name(w3995) -> ("X size (um)"=w4010:sgl, "Z size (um)"=w4009:sgl, "Z-step (nm)"=w3981:dbl)
            n4722 = local write "SW error warning armed"(FALSE ("SW error warning armed")) -> ()
            n4723 = local write "Cycle time array"(u32[] [] ("Cycle time array")) -> ()
            n4724 = local write "Cycle time est offset array"(i16[] [] ("Cycle time array")) -> ()
            n4725 = expression code="x/1e3"(w3981) -> (w4007:dbl)
            n4726 = control-ref of="FIB Image"() -> (w4003:refnum<vi>)
            n4727 = local read "FIB Scan Parameters"() -> (w3994:T32)
            n4728 = local read "FIB Options"() -> (w3993:T33)
            n4729 = shared-variable ".\\Zeiss Library.lvlib\\Milling Z Voltage RT"() -> (w3992:sgl)  [unwired: 1 in, 1 out]
            n4730 = expression code="log2( x/0.1)"(w4010) -> (w4012:sgl)
            n4731 = Round Toward +Infinity(x=w4012) -> (ceil(x): smallest int >= x=w4014:sgl)
            n4732 = Scale By Power Of 2(n=w4014, x=ext 1.0) -> (x*2^n=w4011:ext)
            n4733 = Divide(x=w4009, y=w4007) -> (x/y=w4015:dbl)
            n4734 = Round To Nearest(number=w4015) -> (nearest integer value=w4004:dbl)
            n4735 = local read "Milling para"() -> (w4006:T35)
            n4736 = Increment(x=w4004) -> (x+1=w4005:dbl)
            n4737 = Multiply(x=w4004, y=w4007) -> (x*y=w4008:dbl)
            n4738 = Bundle By Name(cluster=w4006, "X resolution"=w4011, "Z resolution"=w4005, "Z size (um)"=w4008) -> (w3985:T35)
            n4739 = call "FIB image draw milling.vi"("Milling Z Voltage"=w3992, "Milling para"=w3985, "Z offset pre (um)"=w4000, "FIB Options"=w3993, "FIB Scan Parameters"=w3994, "Origin"=w4002, "Image reference"=w4003) -> ("X size factor"=w3983:dbl, "Trapezoidal"=w3982:cluster{"X":i16, "Y":i16}[])  [unwired: 3 in]
            n4740 = local write "Trapezoidal"(w3982) -> ()
            n4741 = control-ref of="Post Image"() -> (w3999:refnum<vi>)
            n4742 = local read "X offset pre (um)"() -> (w3997:dbl)
            n4743 = local read "Y offset pre (um)"() -> (w3996:dbl)
            n4744 = local write "Milling para"(w3985) -> ()
            n4745 = local read "FIB Zoom Parameters"() -> (w3991:T34)
            n4746 = call "FIB zoom image draw milling.vi"("Milling Z voltage"=w3992, "Milling para"=w3985, "Z offset pre (um)"=w3996, "X offset pre (um)"=w3997, "FIB Zoom Parameters"=w3991, "FIB Options"=w3993, "FIB Scan Parameters"=w3994, "Pre image"=FALSE, "Image reference"=w3999) -> ()  [unwired: 3 in]
            n4747 = Unbundle By Name(w3985) -> ("Line milling time (s)"=w3986:sgl, "Lines auto pause"=w3987:u16)
            n4748 = Compound Arithmetic op=MULTIPLY(w3986, w3987, w3983) -> (w3984:dbl)
            n4749 = local write "Milling time (s)"(w3984) -> ()
          }
          event "Milling para.Z-step (nm)": Value Change {
            n4750 = event-data() -> ()  [unwired: 7 out]
            n4751 = local read "Milling para"() -> (w4023:T35)
            n4752 = local read "FIB"() -> (w4024:bool)
            n4753 = case shown="True" w4024 {
              tunnel: [TRUE ("Origin") FALSE ("Origin")] -> w4025
              tunnel: [0.0 ("Y offset pre (um)") w4045] -> w4022
              frame False {
              }
              frame True {
                n4754 = local read "Y offset pre (um)"() -> (w4045:dbl)
              }
            }
            n4755 = Unbundle By Name(w4023) -> ("X size (um)"=w4036:sgl, "Z size (um)"=w4035:sgl, "Z-step (nm)"=w4020:dbl)
            n4756 = expression code="x/1e3"(w4020) -> (w4033:dbl)
            n4757 = control-ref of="FIB Image"() -> (w4029:refnum<vi>)
            n4758 = local read "FIB Scan Parameters"() -> (w4028:T32)
            n4759 = local read "FIB Options"() -> (w4027:T33)
            n4760 = shared-variable ".\\Zeiss Library.lvlib\\Milling Z Voltage RT"() -> (w4026:sgl)  [unwired: 1 in, 1 out]
            n4761 = expression code="log2( x/0.1)"(w4036) -> (w4038:sgl)
            n4762 = Round Toward +Infinity(x=w4038) -> (ceil(x): smallest int >= x=w4040:sgl)
            n4763 = call "FIB image draw milling.vi"("Milling Z Voltage"=w4026, "Milling para"=w4023, "Z offset pre (um)"=w4022, "FIB Options"=w4027, "FIB Scan Parameters"=w4028, "Origin"=w4025, "Image reference"=w4029) -> ()  [unwired: 3 in, 2 out]
            n4764 = Scale By Power Of 2(n=w4040, x=ext 1.0) -> (x*2^n=w4037:ext)
            n4765 = Divide(x=w4035, y=w4033) -> (x/y=w4041:dbl)
            n4766 = Round To Nearest(number=w4041) -> (nearest integer value=w4030:dbl)
            n4767 = local read "Milling para"() -> (w4032:T35)
            n4768 = Increment(x=w4030) -> (x+1=w4031:dbl)
            n4769 = Multiply(x=w4030, y=w4033) -> (x*y=w4034:dbl)
            n4770 = Round To Nearest(number=w4034) -> (nearest integer value=w4021:dbl)
            n4771 = Bundle By Name(cluster=w4032, "X resolution"=w4037, "Z resolution"=w4031, "Z size (um)"=w4021) -> (w4042:T35)
            n4772 = local write "Milling para"(w4042) -> ()
          }
          event "Milling para.Mill start from Last": Value Change {
